vi "Swap_U32.vi"(4 "Swap(T)":bool=TRUE, 6 "b":u32=1, 7 "a":u32=1) -> (1 "b":u32=1, 2 "a":u32=1)   [LabVIEW 2012]
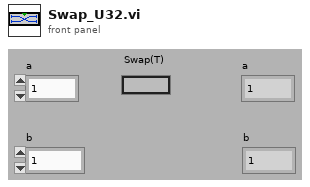
[diagram p1: front panel]
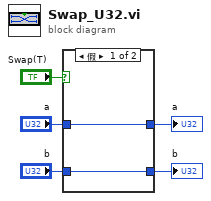
[diagram p0: block diagram]
diagram:
  n1 = case shown="假" "Swap(T)" {
    tunnel: "a" -> [w7 w9]
    tunnel: "b" -> [w6 w8]
    tunnel: [w7 w8] -> w2
    tunnel: [w6 w9] -> w1
    frame False {
    }
    frame True {
    }
  }
  "a" <- w2
  "b" <- w1
